vi "catchProjetsAffect.vi"(2 "Choix":i16(ring) items=["Meuble"], 4 "Id personnel":string) -> (0 "projet_select":string, 1 "size(s)":i32, 3 "liste_projet":string[](array[string]))   [LabVIEW 2024]
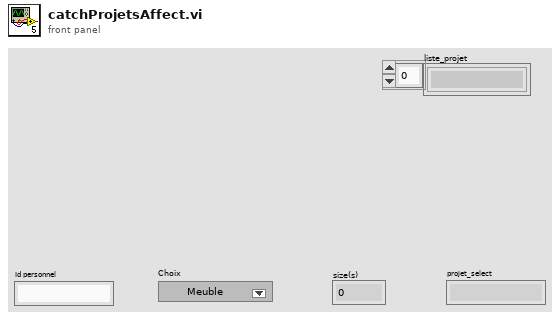
[diagram p1: front panel]
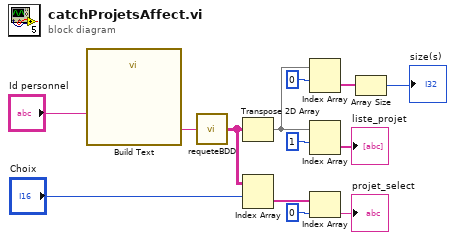
[diagram p0: block diagram]
diagram:
  n1 = call "Build Text"("id"="Id personnel") -> ("Result"=w12:string)  [unwired: 13 in, 1 out]
  n2 = call "requeteBDD.vi"("Requête Sql"=w12) -> ("Table Control"=w2:string[][])
  n3 = Transpose 2D Array(2D array=w2) -> (transposed array=w3:string[][])
  n4 = Index Array(array=w2, index (row)="Choix") -> (element=w10:string[])  [unwired: 1 in]
  n5 = Index Array(array=w3, index (row)=0) -> (element=w6:string[])  [unwired: 1 in]
  n6 = Index Array(array=w3, index (row)=1) -> (element=→"liste_projet":string[])  [unwired: 1 in]
  n7 = Index Array(array=w10, index=0) -> (element=→"projet_select":string)
  n8 = Array Size(array=w6) -> (size(s)=→"size(s)":i32)
